vi "Get Transfer Configuration.vi"(8 "error in (no error)":errorcluster, 11 "Component Configuration in":refnum<class "PXImc Configurations.lvclass">) -> (0 "error out":errorcluster, 1 "Tx Transfer Configuration":refnum<class "Configuration.lvclass">, 2 "Rx Transfer Configuration":refnum<class "Configuration.lvclass">, 3 "Component Configuration out":refnum<class "PXImc Configurations.lvclass">)   [LabVIEW 2017, in "PXImc.lvlib" / "PXImc Configurations.lvclass"]
uses:
  PXImc Configurations.lvclass
  DSF Core.lvlibp/Classes/Configuration/Configuration.lvclass
  Transfer/Transfer Configuration.lvclass
  C:/Git/DSF/Components/DSF Core.lvlibp/Classes/Configuration/Configuration.lvclass
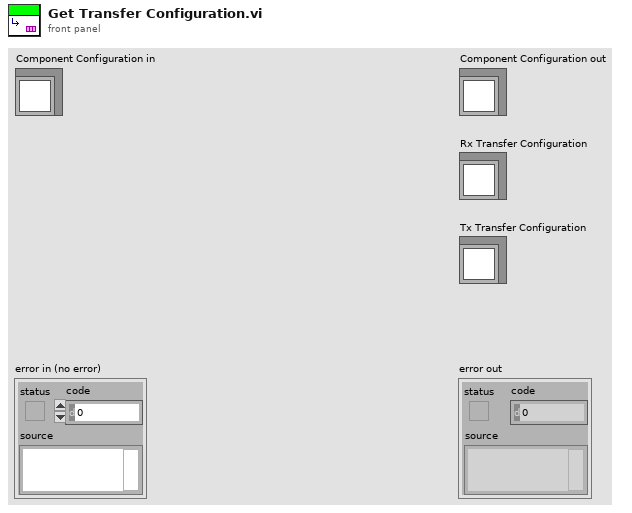
[diagram p1: front panel]
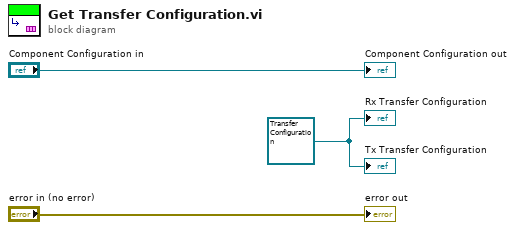
[diagram p0: block diagram]
diagram:
  w1 = refnum<class "Transfer Configuration.lvclass"> refnum ("PXImc.lvlib:PXImc Transfer Configuration")
  "error out" <- "error in (no error)"
  "Component Configuration out" <- "Component Configuration in"
  "Rx Transfer Configuration" <- w1
  "Tx Transfer Configuration" <- w1
